vi "Close.vi"(8 "error in (no error)":errorcluster, 11 "Infiniium in":refnum<class "Infiniium.lvclass">) -> (0 "error out":errorcluster, 3 "Infiniium out":refnum<class "Infiniium.lvclass">)   [LabVIEW 2018, in "ScopePlugins.lvlib" / "Infiniium.lvclass"]
uses:
  Infiniium.lvclass
  C:/Users/ico/Documents/Projects/NistPluggableModules/Scope/ScopePlugins/ScopePluginBaseClass/ScopePluginsBase.lvclass
  ScopePluginBaseClass/ScopePluginsBase.lvclass/ScopePluginsBase.ctl
  ScopePluginBaseClass/Accessors/Read Handle.vi
  ScopePluginBaseClass/Accessors/Read Connected.vi
  <instrlib>/Agilent 90000 Series/Agilent 90000 Series.lvlib
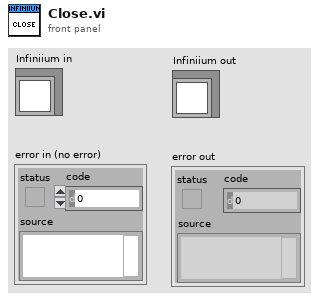
[diagram p1: front panel]
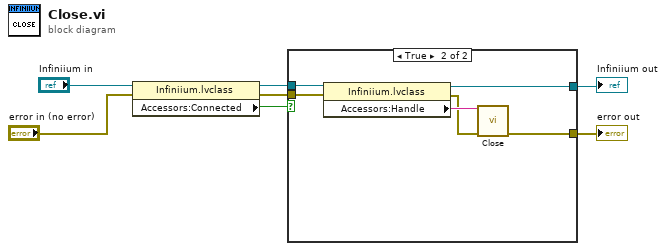
[diagram p0: block diagram]
diagram:
  n1 = property class="Infiniium.lvclass"(reference="Infiniium in", error in="error in (no error)") -> (reference out=w3:refnum<class "Infiniium.lvclass">, error out=w4:errorcluster, "Accessors:Connected"=w5:bool)
  n2 = case shown="True" w5 {
    tunnel: w4 -> [w8 w14]
    tunnel: w3 -> [w9 w15]
    tunnel: [w9 w11] -> w2
    tunnel: [w8 w10] -> w1
    frame False {
    }
    frame True {
      n3 = property class="Infiniium.lvclass"(reference=w15, error in=w14) -> (reference out=w11:refnum<class "Infiniium.lvclass">, error out=w12:errorcluster, "Accessors:Handle"=w13:string)
      n4 = call <instrlib>:"Close.vi"("error in (no error)"=w12, "VISA resource name"=w13) -> ("error out"=w10:errorcluster)  [unwired: 9 in]
    }
  }
  "error out" <- w1
  "Infiniium out" <- w2
